vi "BK Precision 913XX Output DC Volts.vi"() -> ()   [LabVIEW 2012]
doc: "This example shows how to configure the instrument's output voltage level and over voltage protection. The actual voltage level and actual current level are returned."
uses:
  <instrlib>/BK Precision 913XX/BK Precision 913XX.lvlib
panel:
  out "Actual Power Level (W)":dbl format="%.4g"
  out "Actual Voltage Level (V)":dbl format="%.4g"
  out "Actual Current Level (A)":dbl format="%.4g"
  in  "Voltage Limit (36.000 V)":dbl=36.0 min=0.0 max=66.0 step=0.001 format="%.3g"
  in  "Enable OVP (T: Enable)":bool=TRUE
  in  "Channel (1:1)":u16(ring)=1 items=["1"=1, "2"=2, "3"=3]
  in  "Current Limit (0.0 A)":dbl min=0.0 max=25.0 step=1.0 format="%.3f"
  in  "Voltage Level (0.0 V)":dbl format="%.3g"
  in  "Stop Output":bool
  in  "VISA resource name":refnum<visa-resource-name>
  # "(c) 2015 B&K Precision Corporation.  ALL RIGHTS RESERVED."
  # "V"
  # "Over Voltage Protection"
  # "V"
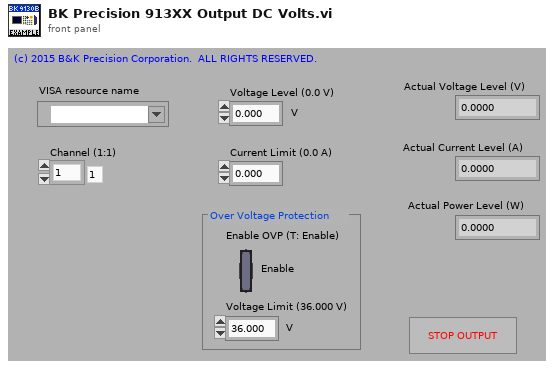
[diagram p1: front panel]
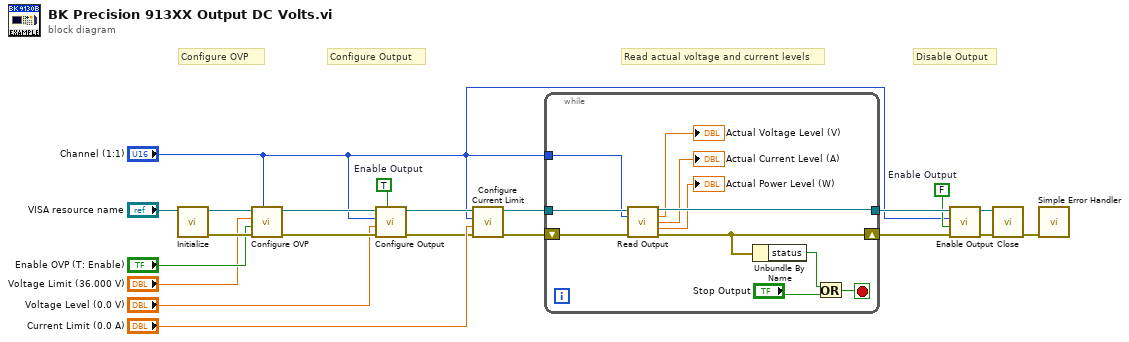
[diagram p0: block diagram]
diagram:
  w2 = FALSE  # Enable Output
  w7 = TRUE  # Enable Output
  # "Disable Output"
  # "Read actual voltage and current levels"
  # "Configure Output"
  # "Configure OVP"
  n1 = call <instrlib>:"Initialize.vi"("VISA resource name"="VISA resource name") -> ("error out"=w19:errorcluster, "VISA resource name out"=w18:refnum<visa-resource-name>)  [unwired: 9 in]
  n2 = call <instrlib>:"Configure OVP.vi"("Channel (1:1)"="Channel (1:1)", "error in (no error)"=w19, "Enable OVP (T: Enable)"="Enable OVP (T: Enable)", "Voltage Limit (36.000 V)"="Voltage Limit (36.000 V)", "VISA resource name"=w18) -> ("error out"=w16:errorcluster, "VISA resource name out"=w17:refnum<visa-resource-name>)  [unwired: 5 in]
  n3 = call <instrlib>:"Configure Output.vi"("Enable Channel Output (F: False)"=w7, "error in (no error)"=w16, "Voltage Level (0.0 V)"="Voltage Level (0.0 V)", "Channel (1:1)"="Channel (1:1)", "VISA resource name"=w17) -> ("error out"=w3:errorcluster, "VISA resource name out"=w4:refnum<visa-resource-name>)  [unwired: 5 in]
  n4 = call <instrlib>:"Configure Current Limit.vi"("error in (no error)"=w3, "Current Limit (0.0 A)"="Current Limit (0.0 A)", "Channel (1:1)"="Channel (1:1)", "VISA resource name"=w4) -> ("error out"=w12:errorcluster, "VISA resource name out"=w11:refnum<visa-resource-name>)  [unwired: 6 in]
  n5 = while {
    tunnel: w11 -> [w29]
    tunnel: [w26] -> w15
    shift-right: [w27] -> w10
    shift-left: w12 -> [w28]
    tunnel: "Channel (1:1)" -> [w22]
    stop <- w32 stop-if-true
    n6 = call <instrlib>:"Read Output.vi"("VISA resource name"=w29, "Channel (1:Channel 1)"=w22, "error in (no error)"=w28) -> ("VISA resource name out"=w26:refnum<visa-resource-name>, "Actual Voltage Level (V)"=→"Actual Voltage Level (V)":dbl, "Actual Current Level (A)"=→"Actual Current Level (A)":dbl, "Actual Power Level (W)"=→"Actual Power Level (W)":dbl, "error out"=w27:errorcluster)  [unwired: 8 in]
    n7 = Unbundle By Name(w27) -> ("status"=w30:bool)
    n8 = Or(x=w30, y="Stop Output") -> (x .or. y?=w32:bool)
  }
  n9 = call <instrlib>:"Enable Output.vi"("error in (no error)"=w10, "Enable Output (F: False)"=w2, "Channel (1:1)"="Channel (1:1)", "VISA resource name"=w15) -> ("error out"=w13:errorcluster, "VISA resource name out"=w14:refnum<visa-resource-name>)  [unwired: 6 in]
  n10 = call <instrlib>:"Close.vi"("error in (no error)"=w13, "VISA resource name"=w14) -> ("error out"=w20:errorcluster)  [unwired: 9 in]
  n11 = call <vilib>:"Simple Error Handler.vi"("error in (no error)"=w20) -> ()  [unwired: 4 in, 5 out]
